vi "CmdConsole.Run.vi"(8 "error in (no error)":errorcluster, 10 "StdOutQ":string, 11 "CmdConsole in":refnum<class "CmdConsole.lvclass">) -> (0 "error out":errorcluster, 2 "Running":bool, 3 "CmdConsole out":refnum<class "CmdConsole.lvclass">)   [LabVIEW 2018, in "CmdConsole.lvclass"]
uses:
  CmdConsole.lvclass
  CmdConsole.lvclass/CmdConsole.ctl
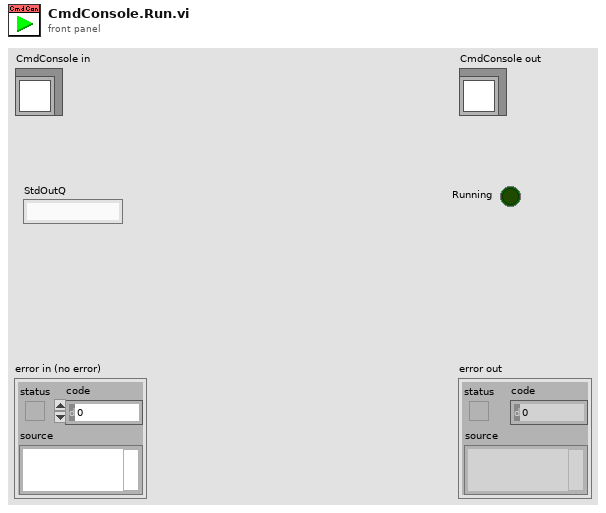
[diagram p1: front panel]
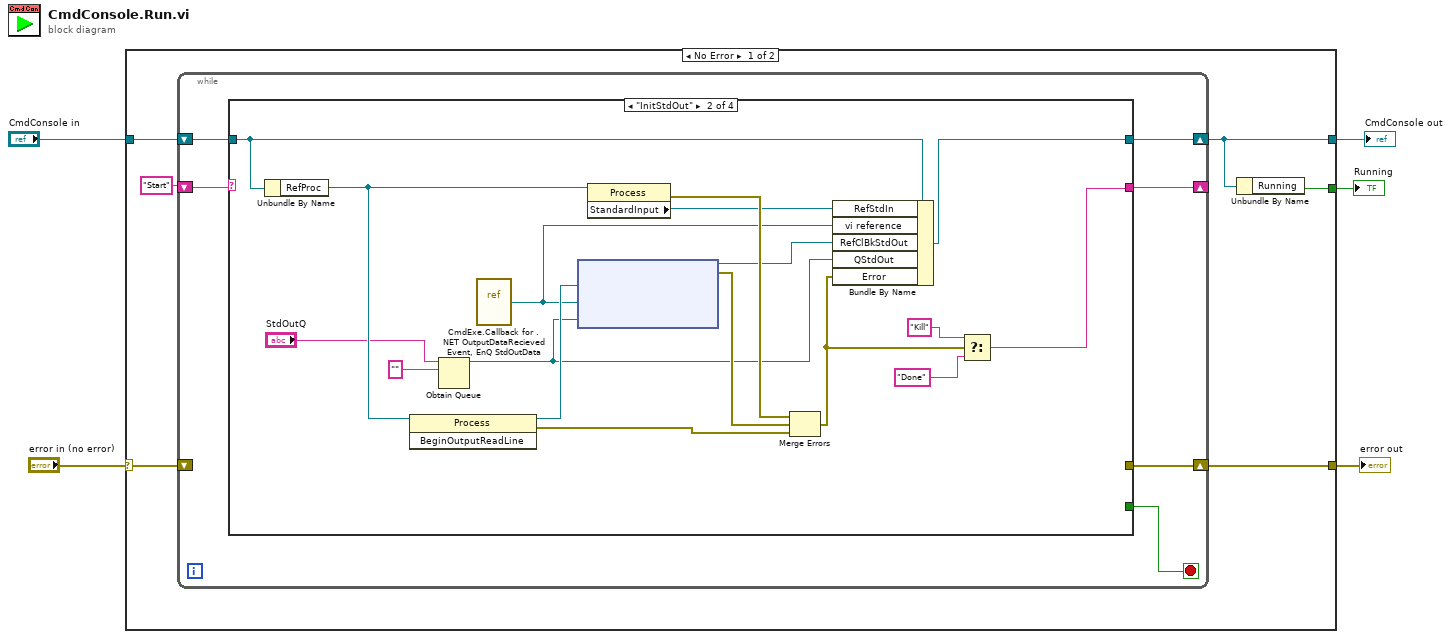
[diagram p0: block diagram]
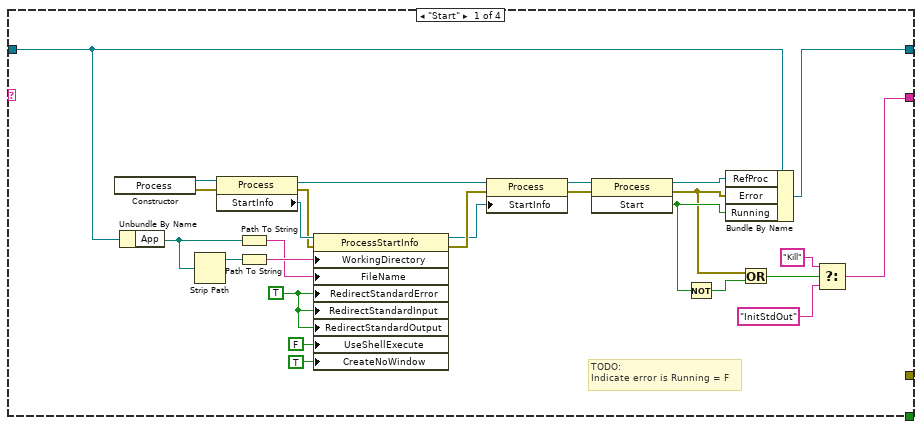
[diagram p2: hidden frame]
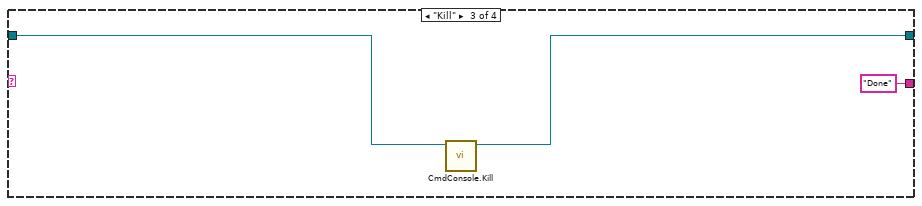
[diagram p3: hidden frame]
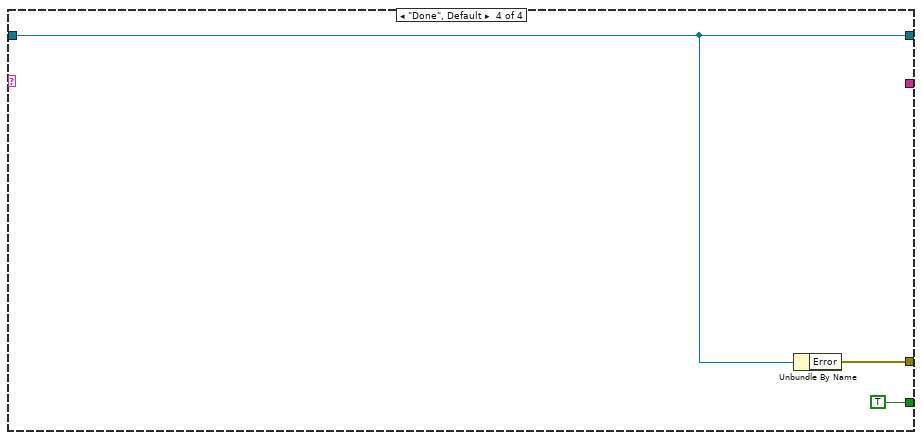
[diagram p4: hidden frame]
diagram:
  n1 = case shown="No Error" "error in (no error)" {
    selector: "error in (no error)" -> [w8 w68]
    tunnel: [w9 w68] -> w4
    tunnel: [w7 w67] -> w2
    tunnel: "CmdConsole in" -> [w11 w67]
    tunnel: [w6 _] -> w1
    frame No Error {
      n2 = while {
        shift-right: [w16] -> w7
        shift-left: w11 -> [w17]
        shift-right: [w14] -> _
        shift-left: "Start" -> [w15]
        shift-right: [w12] -> w9
        shift-left: w8 -> [_]
        stop <- w13 stop-if-true
        n3 = case shown="\"InitStdOut\"" w15 {
          tunnel: w17 -> [w43 w54 w63 w65]
          tunnel: [w26 w52 w61 w65] -> w16
          tunnel: [w18 w46 "Done" _] -> w14
          tunnel: [_ _ _ TRUE] -> w13
          tunnel: [_ _ _ w64] -> w12
          frame "Start" {
            w27 = TRUE ("UseShellExecute")
            # "TODO:\nIndicate error is Running = F"
            n4 = constructor class="Process"() -> (reference out=w42:refnum<k24>, error out=w41:errorcluster)  [unwired: 3 in, 1 out]
            n5 = Unbundle By Name(w43) -> ("App"=w28:path)
            n6 = Strip Path(path=w28) -> (stripped path=w31:path)  [unwired: 1 out]
            n7 = property class="Process"(reference=w42, error in=w41) -> (reference out=w34:refnum<k24>, error out=w35:errorcluster, "StartInfo"=w40:refnum<k24>)
            n8 = Path To String(path=w28) -> (string=w29:string)
            n9 = Path To String(path=w31) -> (string=w30:string)
            n10 = property class="ProcessStartInfo"(reference=w40, error in=w35, "WorkingDirectory"=w30, "FileName"=w29, "RedirectStandardError"=w27, "RedirectStandardInput"=w27, "RedirectStandardOutput"=w27, "UseShellExecute"=FALSE, "CreateNoWindow"=TRUE) -> (reference out=w36:refnum<k24>, error out=w37:errorcluster)
            n11 = property class="Process"(reference=w34, error in=w37, "StartInfo"=w36) -> (reference out=w33:refnum<k24>, error out=w32:errorcluster)
            n12 = invoke class="Process" method="Start"(reference=w33, error in=w32) -> (reference out=w25:refnum<k24>, error out=w22:errorcluster, "Start"=w24:bool)  [unwired: 1 in]
            n13 = Not(x=w24) -> (.not. x?=w23:bool)
            n14 = Bundle By Name(cluster=w43, "RefProc"=w25, "Error"=w22, "Running"=w24) -> (w26:refnum<class "CmdConsole.lvclass">)
            n15 = Or(x=w22, y=w23) -> (x .or. y?=w21:bool)
            n16 = Select(t="Kill", s=w21, f="InitStdOut") -> (s? t:f=w18:string)
          }
          frame "InitStdOut" {
            n17 = Unbundle By Name(w54) -> ("RefProc"=w59:refnum<k24>)
            n18 = invoke class="Process" method="BeginOutputReadLine"(reference=w59) -> (reference out=w60:refnum<k24>, error out=w56:errorcluster)  [unwired: 2 in, 1 out]
            n19 = Obtain Queue(name (unnamed)="StdOutQ", element data type="") -> (queue out=w50:refnum<queue>)  [unwired: 3 in, 2 out]
            n20 = vi-ref "CmdExe.Callback for .NET OutputDataRecieved Event, EnQ StdOutData.vi"() -> ("vi reference"=w44:refnum<vi>)
            n21 = node(w60, w44, w50) -> (w55:refnum<k27>, w57:errorcluster)  [unwired: 2 in]
            n22 = property class="Process"(reference=w59) -> (error out=w58:errorcluster, "StandardInput"=w53:refnum<k24>)  [unwired: 1 in, 1 out]
            n23 = Merge Errors(w58, w57, w56) -> (w49:errorcluster)
            n24 = Bundle By Name(cluster=w54, "RefStdIn"=w53, "vi reference"=w44, "RefClBkStdOut"=w55, "QStdOut"=w50, "Error"=w49) -> (w52:refnum<class "CmdConsole.lvclass">)
            n25 = Select(t="Kill", s=w49, f="Done") -> (s? t:f=w46:string)
          }
          frame "Kill" {
            n26 = call "CmdConsole.Kill.vi"("CmdConsole in"=w63) -> ("CmdConsole out"=w61:refnum<class "CmdConsole.lvclass">)  [unwired: 9 in, 1 out]
          }
          frame "Done", Default {
            n27 = Unbundle By Name(w65) -> ("Error"=w64:errorcluster)
          }
        }
      }
      n28 = Unbundle By Name(w7) -> ("Running"=w6:bool)
    }
    frame Error {
    }
  }
  "error out" <- w4
  "CmdConsole out" <- w2
  "Running" <- w1
